vi "simple_examples.vi"() -> ()   [LabVIEW 2018, in "LV-0mq-Julia_roundtrip-lib.lvlib" / "LV2Julia_examples.lvlib"]
uses:
  LV2Julia_examples.lvlib
  LV2Julia_core/VIs/Server or client state.ctl
  LV2Julia_core/VIs/detailed error info.ctl
  LV2Julia_core/VIs/StackFrame.ctl
  simple examples functions.ctl
  LV2Julia_core/VIs/Commands.ctl
  edf81fa3-46bf-427f-9605-85b461656974.vi
  29886417-d43f-41fb-9c0c-469db3f8c96d.vi
  3fe35f36-217a-40a5-a789-8326c52a1f5c.vi
  35a44a82-786b-41ea-be73-9a4468e4df9d.vi
  edf81fa3-46bf-427f-9605-85b461656974.vi/d78438c1-e9c2-4049-8a01-ea359766d27e.vi
  29886417-d43f-41fb-9c0c-469db3f8c96d.vi/726a0e03-44e9-4b5b-8c33-3fdb3adf96f2.vi
  3fe35f36-217a-40a5-a789-8326c52a1f5c.vi/be66880e-2f9f-43fa-8a25-3020ddce25df.vi
  35a44a82-786b-41ea-be73-9a4468e4df9d.vi/e765cad0-9840-4168-a112-da73896eb643.vi
  35a44a82-786b-41ea-be73-9a4468e4df9d.vi/f3238023-a8b3-435f-be8b-4be774610aa1.vi
  edf81fa3-46bf-427f-9605-85b461656974.vi/d78438c1-e9c2-4049-8a01-ea359766d27e.vi/edf13171-bb8c-4b0e-8a13-cfaee6010a46.vi
  29886417-d43f-41fb-9c0c-469db3f8c96d.vi/726a0e03-44e9-4b5b-8c33-3fdb3adf96f2.vi/e7bf7d0e-5fa3-492d-91d8-494ec4c78bd1.vi
  29886417-d43f-41fb-9c0c-469db3f8c96d.vi/726a0e03-44e9-4b5b-8c33-3fdb3adf96f2.vi/bcfacdb4-d734-4844-97c1-59f988d0ab4b.vi
  29886417-d43f-41fb-9c0c-469db3f8c96d.vi/726a0e03-44e9-4b5b-8c33-3fdb3adf96f2.vi/27f03db2-f0c9-44fc-95a3-84f8622bf8b3.vi
  3fe35f36-217a-40a5-a789-8326c52a1f5c.vi/be66880e-2f9f-43fa-8a25-3020ddce25df.vi/b22e8afe-8408-4b96-ba33-df0573f8bda9.vi
  3fe35f36-217a-40a5-a789-8326c52a1f5c.vi/be66880e-2f9f-43fa-8a25-3020ddce25df.vi/973810d6-8273-42e9-becd-a912c4fb1f62.vi
  3fe35f36-217a-40a5-a789-8326c52a1f5c.vi/be66880e-2f9f-43fa-8a25-3020ddce25df.vi/742d8af4-4bb6-4e08-85d7-281a839dc2ce.vi
  35a44a82-786b-41ea-be73-9a4468e4df9d.vi/e765cad0-9840-4168-a112-da73896eb643.vi/dc34fd2d-f794-448f-aba6-043ae9d4d40f.vi
  35a44a82-786b-41ea-be73-9a4468e4df9d.vi/e765cad0-9840-4168-a112-da73896eb643.vi/fa03b5a1-01ca-4e07-872a-a6bd434a2e33.vi
  edf81fa3-46bf-427f-9605-85b461656974.vi/d78438c1-e9c2-4049-8a01-ea359766d27e.vi/edf13171-bb8c-4b0e-8a13-cfaee6010a46.vi/3952a552-d88b-4b70-b2de-8936c03ae8d7.vi
  35a44a82-786b-41ea-be73-9a4468e4df9d.vi/e765cad0-9840-4168-a112-da73896eb643.vi/dc34fd2d-f794-448f-aba6-043ae9d4d40f.vi/6b1990a7-d1b9-4824-acae-e43fafbf4c5e.vi
  LV2Julia_core/VIs/jl-scripts path.vi
  LV2Julia_core/VIs/check ID validity.vi
  LV2Julia_core/VIs/bindata_descr to JSON.vi
  LV2Julia_core/VIs/check cluster field names.vi
  LV2Julia_core/VIs/concat JSON.vi
  LV2Julia_core/VIs/build request.vi
  LV2Julia_core/VIs/Parse server response.vi
  LV2Julia_core/VIs/log jl exceptions.vi
  <vilib>/Utility/error.llb/Error Cluster From Error Code.vi
  LV2Julia_core/LV2Julia_core.lvlib
  <vilib>/measure/NI_MABase.lvlib
panel:
  out "ZMQ timeout":bool
  out "Julia script file path":path
  out "temporary script path":path
  out "Jl Server state":T1
  in  "execution control pages":enum32{"Start", "go - test"}(tab)
  in  "go":bool caption="go (Julia Server started externally)"
  in  "Start with Julia":bool caption="Start Julia Server and go"
  in  "ZMQ endpoint":string="tcp://127.0.0.1:5555"
  in  "p":dbl=1.0
  in  "fn":T2 caption="select function at Server" items=["arr_amplitude", "arr_length", "arr_mean", "arr_median", "arr_rms", "vec_amplify", "vec_attenuate", "vec_power"]
  in  "trim @ begin":dbl
  in  "trim @ end":dbl
  in  "Group":T3(tab)
  out "Server response":dbl
  out "data received plot":dbl[](graph)
  out "data received":dbl[](array[numeric]) format="%.3f"
  out "RMS":dbl
  out "detailed error info":T4
  out "current error":errorcluster
  out "final error":errorcluster
  out "short err code":u8
  in  "tones":T6(array[cluster])=[{"frequency"=10.0, "amplitude"=1.0, "phase"=0.0}, {"frequency"=20.0, "amplitude"=0.1, "phase"=0.0}] {"phase" format="%.2p"; "amplitude" format="%0.2p"; "frequency" format="%0.2p"}
  in  "noise (rms)":dbl=0.1 format="%.2p"
  in  "offset":dbl format="%.2p"
  in  "sampling info":cluster{"Fs":dbl, "#s":dbl}={"Fs"=1000.0, "#s"=1000.0} {"Fs" format="%.2p"}
  in  "next":bool
  out "data sent to server":dbl[](graph)
  out "data sent":dbl[](array[numeric]) format="%.3f"
  out "function name":string
  in  "stop this VI only":bool
  in  "stop both this VI and Julia Server":bool
  # "tcp://127.0.0.1:5555 \nfor local Julia Server\n\nFor a Julia Server running on a separate computer,  you probably must use an IPv4 address in numeric form (not a DNS name) - see https://stackoverflow.com/questions/6024003/why-doesnt-zeromq-work-on-localhost.\n\nThis control only used if Julia Server is not being started by this VI."
  # "generate sample array"
  # "function and parameter"
  # "enter a negative or a large positive value to cause an exception"
  # "data returned by server"
  # "data sent to server"
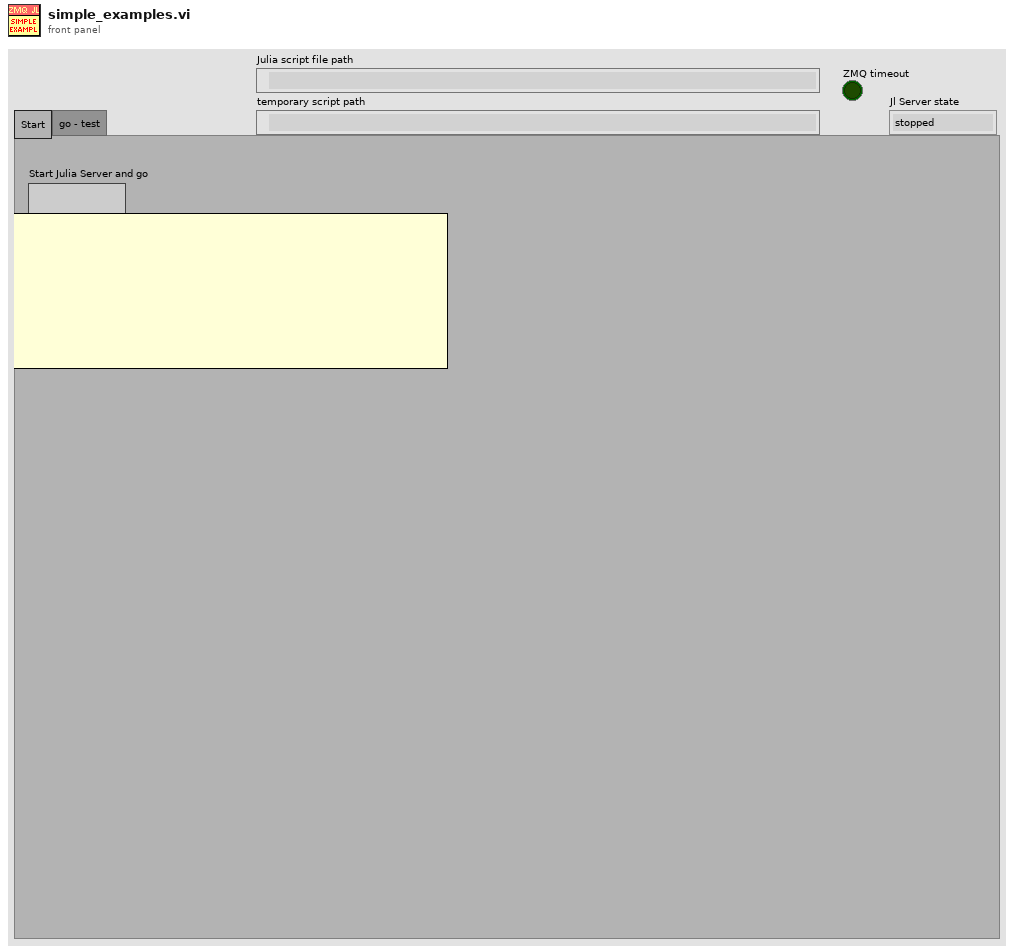
[diagram p1: front panel]
types:
  T1 = typedef "LV-0mq-Julia_roundtrip-lib.lvlib/LV2Julia_core.lvlib/Server or client state.ctl" = enum16{"stopped", "running", "unknown"}
  T2 = typedef "LV-0mq-Julia_roundtrip-lib.lvlib/LV2Julia_examples.lvlib/simple examples functions.ctl" = u16
  T3 = enum32{"fns returning scalar", "fns returning vector", "error"}
  T4 = typedef "LV-0mq-Julia_roundtrip-lib.lvlib/LV2Julia_core.lvlib/detailed error info.ctl" = cluster{"exception_or_info":string, "trace":T5[]}
  T5 = typedef "LV-0mq-Julia_roundtrip-lib.lvlib/LV2Julia_core.lvlib/StackFrame.ctl" = cluster{"frame_summary":string, "func":string, "linfo":string, "file":string, "line":i32, "pointer":u64, "from_c":bool, "inlined":bool}
  T6 = cluster{"frequency":dbl, "amplitude":dbl, "phase":dbl}[]
  T7 = typedef "LV-0mq-Julia_roundtrip-lib.lvlib/LV2Julia_core.lvlib/Commands.ctl" = enum16{"Start Jl-server & Init LV-client", "Send request & Get response ", "Stop Jl-server & Cleanup LV-client", "Cleanup LV-client", "Start Jl-server", "Stop Jl-server", "Init LV-Client", "Cleanup LV-Client", "(not allowed)", "Set LV Client state", "Set Jl Server state", "set ZMQ timeout", "read ZMQ timeout", "read-out state"}
  T8 = enum8{"Enabled", "Disabled", "Disabled and Grayed Out"}
  T9 = typedef "LV-0mq-Julia_roundtrip-lib.lvlib/LV2Julia_core.lvlib/Bindata&description.ctl" = cluster{"bindata_descr":T10[], "bindata":u8[]}
  T10 = typedef "LV-0mq-Julia_roundtrip-lib.lvlib/LV2Julia_core.lvlib/Bindata description.ctl" = cluster{"nofbytes":i32, "numtype":string, "start":i32, "arrdims":i32[], "kwarg_name":string, "category":string}
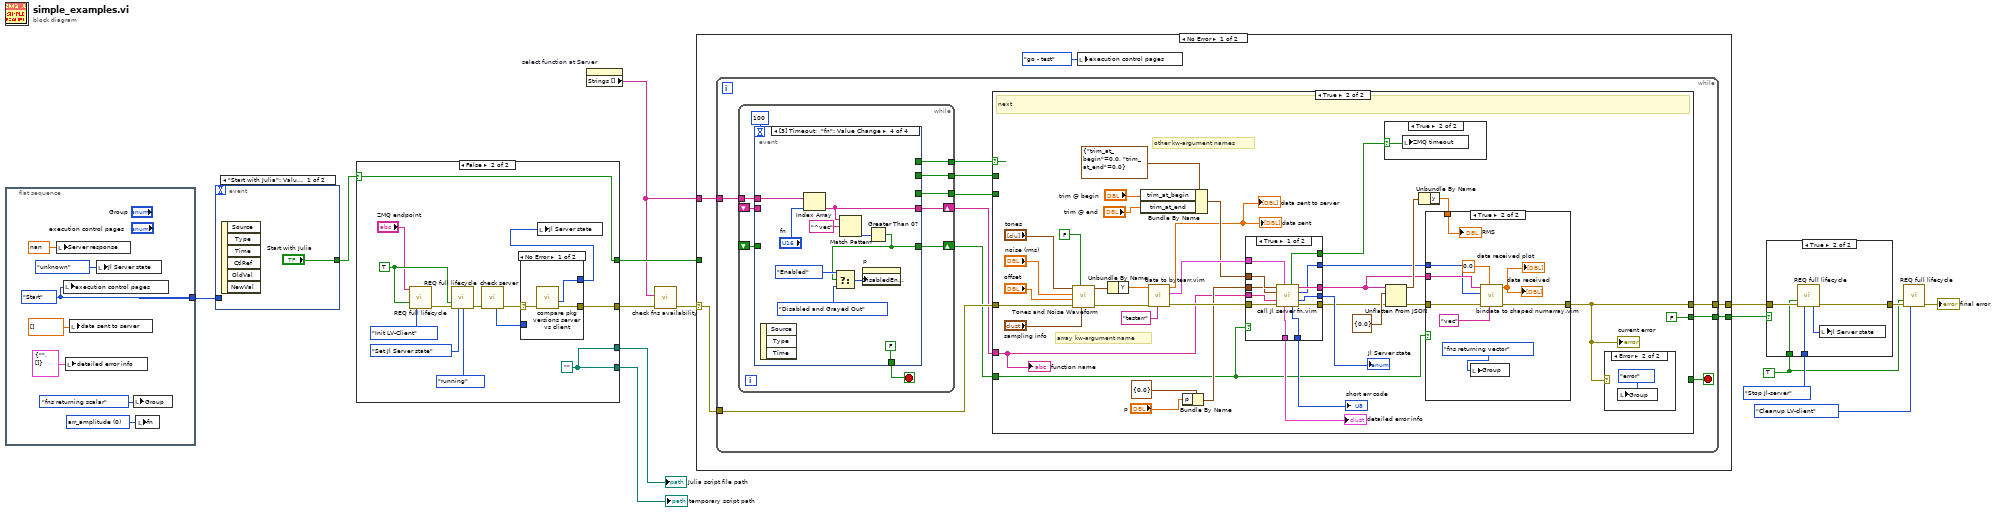
[diagram p0: block diagram]
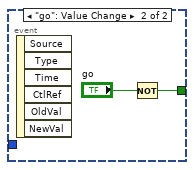
[diagram p2: hidden frame]
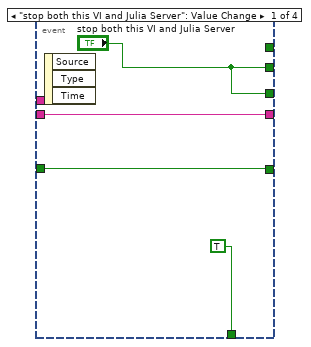
[diagram p3: hidden frame]
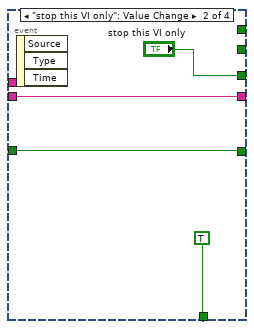
[diagram p4: hidden frame]
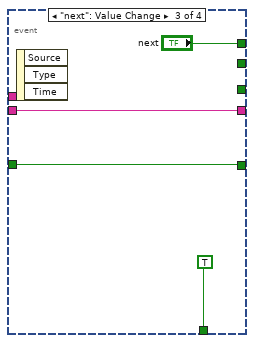
[diagram p5: hidden frame]
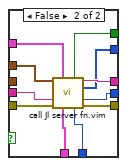
[diagram p7: hidden frame]
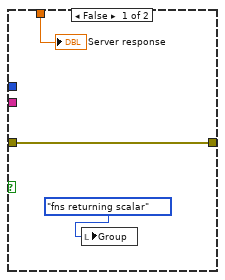
[diagram p9: hidden frame]
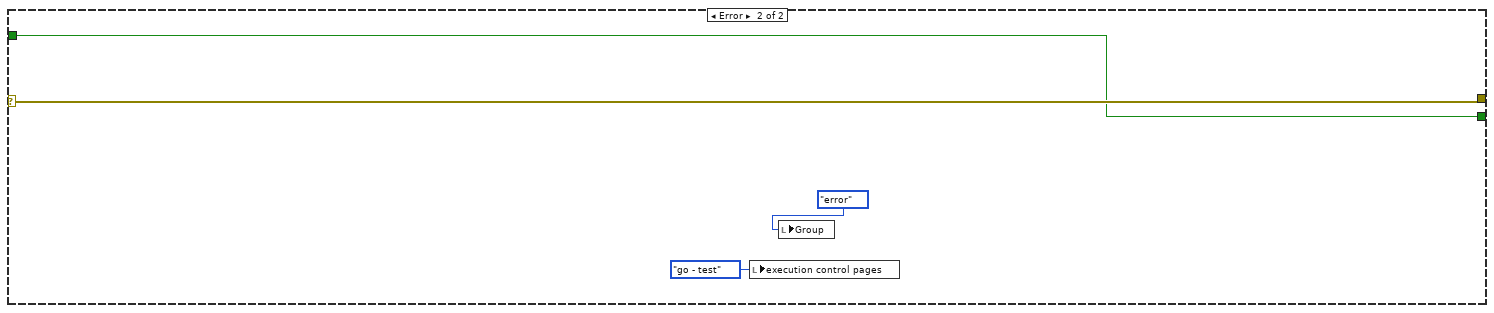
[diagram p11: hidden frame]
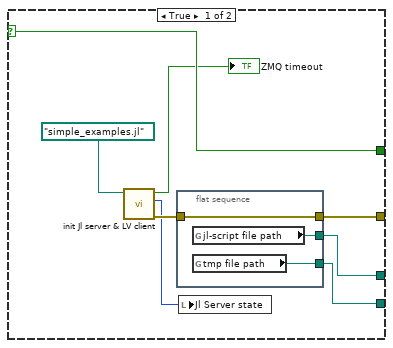
[diagram p12: hidden frame]
diagram:
  w10 = TRUE ("Force command")
  n1 = flat-sequence {
    tunnel: [w22] -> w6
    frame #0 {
      w16 = T2 0 items=["arr_amplitude", "arr_length", "arr_mean", "arr_median", "arr_rms", "vec_amplify", "vec_attenuate", "vec_power"] ("fn")
      w22 = enum32{"Start", "go - test", "finish"}."Start" ("execution control pages")
      n2 = local write "Server response"(nan ("Server response")) -> ()
      n3 = local write "execution control pages"(w22) -> ()
      n4 = local write "detailed error info"(T4 {"exception_or_info"="", "trace"=[]} ("detailed error info")) -> ()
      n5 = local write "data sent to server"(dbl[] []) -> ()
      n6 = local write "Jl Server state"(Server_or_client_state."unknown" ("Jl Server state out")) -> ()
      n7 = local write "Group"(T3."fns returning scalar" ("Group")) -> ()
      n8 = local write "fn"(w16) -> ()
    }
  }
  n9 = event shown="[0] \"Start with Julia\": Value Change" {
    selector: _ -> [_ _]
    dyn-events: _ -> [_ _]
    timeout: _ -> [_ _]
    tunnel: ["Start with Julia" w24] -> w8
    tunnel: w6 -> [_ _]
    event "Start with Julia": Value Change {
      n10 = event-data() -> ()  [unwired: 1 in, 6 out]
    }
    event "go": Value Change {
      n11 = event-data() -> ()  [unwired: 1 in, 6 out]
      n12 = Not(x="go") -> (.not. x?=w24:bool)
    }
  }
  n13 = case shown="False" w8 {
    selector: w8 -> [w33 w45]
    tunnel: [w32 w39] -> w5
    tunnel: [w33 w45] -> w7
    tunnel: [w31 w42] -> w1
    tunnel: [w30 w42] -> w2
    frame True {
      n14 = call "init Jl server & LV client.vi"("Julia user functions script"=path "simple_examples.jl") -> ("error out"=w27:errorcluster, "Jl Server state out"=w26:T1, "timeout?"=→"ZMQ timeout":bool)  [unwired: 8 in]
      n15 = flat-sequence {
        tunnel: [w36] -> w32
        tunnel: w27 -> [w36]
        tunnel: [w35] -> w31
        tunnel: [w34] -> w30
        frame #0 {
          n16 = global read "jl-scripts path.vi" "jl-script file path"() -> (w35:path)
          n17 = global read "jl-scripts path.vi" "tmp file path"() -> (w34:path)
        }
      }
      n18 = local write "Jl Server state"(w26) -> ()
    }
    frame False {
      w42 = path ""
      w47 = TRUE ("Force command")
      n19 = call "REQ full lifecycle.vi"("ZMQ endpoint"="ZMQ endpoint", "Force command"=w47, "command"=Commands."Init LV-Client") -> ("error out"=w44:errorcluster)  [unwired: 6 in, 6 out]
      n20 = call "REQ full lifecycle.vi"("Force command"=w47, "error in"=w44, "command"=Commands."Set Jl Server state", "Jl Server state in"=Server_or_client_state."running") -> ("error out"=w43:errorcluster)  [unwired: 5 in, 6 out]
      n21 = call "check server.vi"("error in"=w43) -> ("error out"=w40:errorcluster, "Jl Server state out"=w38:T1)  [unwired: 6 in, 3 out]
      n22 = case shown="No Error" w40 {
        selector: w40 -> [w52 w54]
        tunnel: [w51 w54] -> w39
        tunnel: [w50 w53] -> w37
        tunnel: w38 -> [_ w53]
        frame No Error {
          n23 = call "compare pkg versions server vs client.vi"("error in (no error)"=w52) -> ("error out"=w51:errorcluster, "Jl Server state out"=w50:T1)  [unwired: 4 in, 5 out]
        }
        frame Error {
        }
      }
      n24 = local write "Jl Server state"(w37) -> ()
    }
  }
  "temporary script path" <- w2
  "Julia script file path" <- w1
  n25 = property on="select function at Server" class="Ring (strict)"() -> ("Strings []"=w3:string[])  [unwired: 2 in, 2 out]
  n26 = call "check fns availability.vi"("error in (no error)"=w5, "fns list is"=w3) -> ("error out"=w4:errorcluster)  [unwired: 3 in, 6 out]
  n27 = case shown="No Error" w4 {
    selector: w4 -> [w58 w180]
    tunnel: [w59 w180] -> w15
    tunnel: [w57 w179] -> w9
    tunnel: w3 -> [w56 _]
    tunnel: w7 -> [_ w179]
    frame No Error {
      n28 = while {
        tunnel: w58 -> [w68]
        tunnel: [w69] -> w59
        tunnel: [w65] -> w57
        tunnel: w56 -> [w63]
        stop <- w66 stop-if-true
        n29 = while {
          tunnel: [w79] -> w67
          tunnel: [w78] -> w64
          tunnel: w63 -> [w75]
          shift-right: [w74] -> w62
          shift-left: _ -> [w71]
          shift-right: [w73] -> w61
          shift-left: _ -> [w72]
          tunnel: [w70] -> w60
          stop <- w77 stop-if-true
          n30 = event shown="[3] Timeout;  \"fn\": Value Change" {
            selector: _ -> [_ _ _ _]
            dyn-events: _ -> [_ _ _ _]
            timeout: 100 -> [_ _ _ _]
            tunnel: ["stop both this VI and Julia Server" _ _ _] -> w78
            tunnel: [_ _ "next" _] -> w79
            tunnel: [TRUE TRUE TRUE FALSE] -> w77
            tunnel: w75 -> [_ _ _ w95]
            tunnel: [w81 w85 w89 w94] -> w74
            tunnel: [w82 w86 w88 w93] -> w73
            tunnel: w72 -> [w82 w86 w88 _]
            tunnel: w71 -> [w81 w85 w89 _]
            tunnel: ["stop both this VI and Julia Server" "stop this VI only" _ _] -> w70
            event "stop both this VI and Julia Server": Value Change {
              n31 = event-data() -> ()  [unwired: 1 in, 3 out]
            }
            event "stop this VI only": Value Change {
              n32 = event-data() -> ()  [unwired: 1 in, 3 out]
            }
            event "next": Value Change {
              n33 = event-data() -> ()  [unwired: 1 in, 3 out]
            }
            event Timeout; Value Change {
              n34 = event-data() -> ()  [unwired: 1 in, 3 out]
              n35 = Index Array(array=w95, index="fn") -> (element=w93:string)
              n36 = Match Pattern(string=w93, regular expression="^vec") -> (offset past match=w99:i32)  [unwired: 1 in, 3 out]
              n37 = Greater Than 0?(x=w99) -> (x > 0?=w94:bool)
              n38 = Select(t=T8."Enabled" ("Disabled"), s=w94, f=T8."Disabled and Grayed Out" ("Disabled")) -> (s? t:f=w101:T8)
              n39 = property on="p" class="DigNum (strict)"("DisabledEnum"=w101) -> ()  [unwired: 2 in, 2 out]
            }
          }
        }
        n40 = case shown="True" w67 {
          tunnel: [w104 w120] -> w69
          tunnel: w68 -> [w104 w125]
          tunnel: [w103 w124] -> w66
          tunnel: w60 -> [w103 _]
          tunnel: [w102 w124] -> w65
          tunnel: w64 -> [w102 _]
          tunnel: w62 -> [_ w106]
          tunnel: w61 -> [_ w108]
          frame False {
            # "stop"
          }
          frame True {
            w124 = FALSE ("stop this VI only")
            # "other kw-argument names"
            # "array kw-argument name"
            # "next"
            n41 = call <vilib>:"Tones and Noise Waveform.vi"("sampling info"="sampling info", "reset signal"=FALSE, "error in (no error)"=w125, "offset"="offset", "noise (rms)"="noise (rms)", "tones"="tones") -> ("error out"=w126:errorcluster, "signal out"=w132:waveform(dbl))  [unwired: 4 in]
            n42 = Unbundle By Name(w132) -> ("Y"=w127:dbl[])
            n43 = Bundle By Name(cluster=cluster{"trim_at_begin":dbl, "trim_at_end":dbl} {"trim_at_begin"=0.0, "trim_at_end"=0.0}, "trim_at_begin"="trim @ begin", "trim_at_end"="trim @ end") -> (w110:cluster{"trim_at_begin":dbl, "trim_at_end":dbl})
            n44 = call "data to bytearr.vim"("kwarg_name"="testarr", "error in (no error)"=w126, "data in"=w127) -> ("error out"=w118:errorcluster, "Bindata & descr out"=w111:T9, "flattened data out"=→"data sent" →"data sent to server":dbl[])  [unwired: 6 in]
            n45 = Bundle By Name(cluster=cluster{"p":dbl} {"p"=0.0}, "p"="p") -> (w109:cluster{"p":dbl})
            n46 = case shown="True" w106 {
              tunnel: w118 -> [w151 w162]
              tunnel: [w150 w161] -> w117
              tunnel: [w149 w160] -> w116
              tunnel: [w148 w159] -> w115
              tunnel: [w147 w158] -> w114
              tunnel: [w146 w157] -> w113
              tunnel: [w145 w156] -> w112
              tunnel: w111 -> [w144 w155]
              tunnel: w110 -> [w143 w154]
              tunnel: w109 -> [w142 _]
              tunnel: w108 -> [w141 w153]
              tunnel: [w140 w152] -> w107
              frame True {
                n47 = call "call Jl server fn.vim"("Arguments 1"=w143, "Bindata & descr in"=w144, "Arguments 2"=w142, "fun2call"=w141, "error in (no error)"=w151) -> ("timeout?"=w145:bool, "JSON received"=w147:string, "binary data received"=w146:u8[], "Jl Server state out"=w149:T1, "detailed error info"=w150:T4, "return code"=w140:u8, "error out"=w148:errorcluster)  [unwired: 4 in]
              }
              frame False {
                n48 = call "call Jl server fn.vim"("Arguments 1"=w154, "Bindata & descr in"=w155, "fun2call"=w153, "error in (no error)"=w162) -> ("timeout?"=w156:bool, "JSON received"=w158:string, "binary data received"=w157:u8[], "Jl Server state out"=w160:T1, "detailed error info"=w161:T4, "return code"=w152:u8, "error out"=w159:errorcluster)  [unwired: 5 in]
              }
            }
            "short err code" <- w107
            "Jl Server state" <- w116
            "detailed error info" <- w117
            n49 = case shown="True" w112 {
              selector: w112 -> [_ w163]
              frame False {
              }
              frame True {
                n50 = local write "ZMQ timeout"(w163) -> ()
              }
            }
            n51 = Unflatten From JSON(JSON string=w114, type and defaults=cluster{"y":dbl} {"y"=0.0} ("parsed response"), error in (no error)=w115) -> (value=w138:cluster{"y":dbl}, error out=w121:errorcluster)  [unwired: 4 in]
            n52 = Unbundle By Name(w138) -> ("y"=w119:dbl)
            n53 = case shown="True" w106 {
              tunnel: w121 -> [w166 w174]
              tunnel: [w166 w173] -> w120
              tunnel: w113 -> [_ w167]
              tunnel: w114 -> [_ w168]
              tunnel: w119 -> [w164 w170]
              frame False {
                n54 = local write "Group"(T3."fns returning scalar" ("Group")) -> ()
                "Server response" <- w164
              }
              frame True {
                n55 = local write "Group"(T3."fns returning vector" ("Group")) -> ()
                n56 = call "bindata to shaped numarray.vim"("name"="vec" ("kwarg_name"), "element type"=0.0 ("data type"), "error in (no error)"=w174, "binary data"=w167, "JSON in"=w168) -> ("error out"=w173:errorcluster, "numarray 1D"=→"data received plot" →"data received":dbl[])  [unwired: 3 in, 2 out]
                "RMS" <- w170
              }
            }
            "current error" <- w120
            n57 = case shown="Error" w120 {
              frame No Error {
              }
              frame Error {
                n58 = local write "Group"(T3."error" ("Group")) -> ()
              }
            }
            "function name" <- w108
          }
        }
      }
      n59 = local write "execution control pages"(enum32{"Start", "go - test", "finish"}."go - test" ("execution control pages")) -> ()
    }
    frame Error {
      n60 = local write "execution control pages"(enum32{"Start", "go - test", "finish"}."go - test" ("execution control pages")) -> ()
      n61 = local write "Group"(T3."error" ("Group")) -> ()
    }
  }
  n62 = case shown="True" w9 {
    tunnel: w15 -> [w181 w186]
    tunnel: Commands."Stop Jl-server" ("command") -> [_ w185]
    tunnel: [w181 w184] -> w13
    tunnel: w10 -> [_ w183]
    frame False {
    }
    frame True {
      n63 = call "REQ full lifecycle.vi"("Force command"=w183, "error in"=w186, "command"=w185) -> ("Jl Server state out"=w182:T1, "error out"=w184:errorcluster)  [unwired: 6 in, 5 out]
      n64 = local write "Jl Server state"(w182) -> ()
    }
  }
  n65 = call "REQ full lifecycle.vi"("Force command"=w10, "error in"=w13, "command"=Commands."Cleanup LV-client") -> ("error out"=→"final error":errorcluster)  [unwired: 6 in, 6 out]
